vi "Preview Next Msg.vi"(8 "error in":errorcluster, 9 "Termination (Exit)":string="Exit", 10 "timeout (0ms)":i32, 11 "Msg Queue In":refnum<queue>) -> (0 "error out":errorcluster, 1 "Msg Value":variant, 2 "Msg Name":string, 3 "Msg Queue Out":refnum<queue>, 4 "Stop?":bool, 5 "timed out?":bool, 6 "Q Backlog":i32)   [LabVIEW 2018, in "EZ Message.lvlib"]
uses:
  EZ Message.lvlib
  Message.ctl
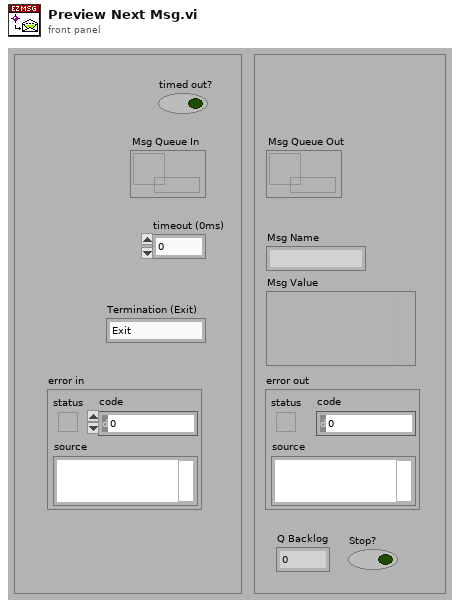
[diagram p1: front panel]
types:
  T1 = typedef "EZ Message.lvlib/Message.ctl" = cluster{"Name":string, "Value":variant}
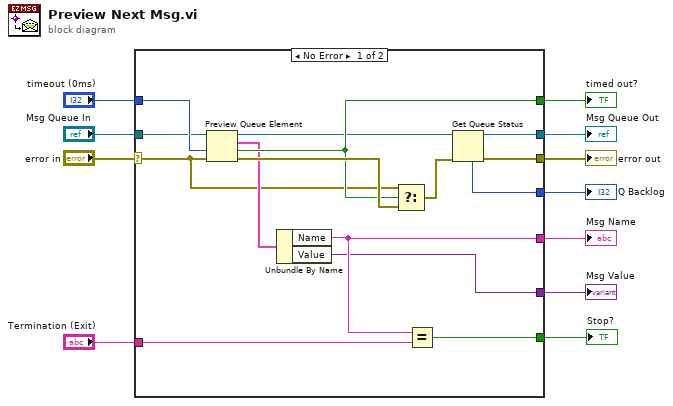
[diagram p0: block diagram]
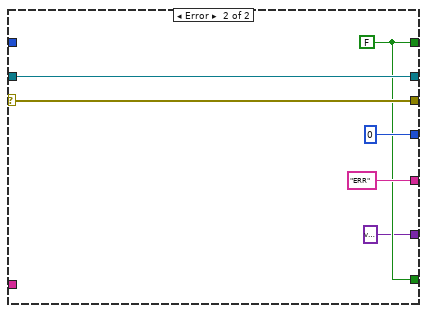
[diagram p2: hidden frame]
diagram:
  n1 = case shown="No Error" "error in" {
    selector: "error in" -> [w12 w32]
    tunnel: [w26 w28] -> w11
    tunnel: [w25 "ERR" ("Name")] -> w10
    tunnel: "Termination (Exit)" -> [w24 _]
    tunnel: [w21 w28] -> w8
    tunnel: [w20 w31] -> w7
    tunnel: [w19 w32] -> w6
    tunnel: [w18 variant ("Value")] -> w1
    tunnel: [w17 0 ("# elements in queue")] -> w5
    tunnel: "timeout (0ms)" -> [w15 _]
    tunnel: "Msg Queue In" -> [w14 w31]
    frame No Error {
      n2 = Preview Queue Element(queue=w14, timeout in ms (-1)=w15, error in (no error)=w12) -> (queue out=w13:refnum<queue>, element=w16:T1, timed out?=w21:bool, error out=w22:errorcluster)
      n3 = Unbundle By Name(w16) -> ("Name"=w25:string, "Value"=w18:variant)
      n4 = Select(t=w12, s=w21, f=w22) -> (s? t:f=w23:errorcluster)
      n5 = Equal?(x=w25, y=w24) -> (x = y?=w26:bool)
      n6 = Get Queue Status(queue=w13, error in (no error)=w23) -> (queue out=w20:refnum<queue>, error out=w19:errorcluster, # elements in queue=w17:i32)  [unwired: 1 in, 5 out]
    }
    frame Error {
      w28 = FALSE ("timed out?")
    }
  }
  "Stop?" <- w11
  "Msg Name" <- w10
  "timed out?" <- w8
  "Msg Queue Out" <- w7
  "error out" <- w6
  "Q Backlog" <- w5
  "Msg Value" <- w1
